vi "ActionVIOnCompile.vi"(8 "error in (no error)":errorcluster, 11 "Device Item Ref in":T1 format="%.0x") -> (0 "error out":errorcluster)   [LabVIEW 2021, in "FPGA Addon System Explorer.lvlib"]
uses:
  FPGA Addon System Explorer.lvlib
  <vilib>/NI VeriStand/Custom Device API/Custom Device Item Ref.ctl
  <vilib>/NI VeriStand/Custom Device API/Data Access Type.ctl
  Addon Shared/Types/FG Action.ctl
  Addon Shared/Types/Compiled.Settings.ctl
  Addon Shared/Types/Compiled.RegisterSettings.ctl
  Addon Shared/Types/Scalar Type.ctl
  Addon Shared/Types/Register Information.ctl
  Addon Shared/Types/FPGA Addon Data Type.ctl
  <vilib>/NI VeriStand/Custom Device API/Block Data Reference.ctl
  <vilib>/NI VeriStand/Custom Device API/Data Reference.ctl
  Addon Shared/Types/Compiled.DMASettings.ctl
  Addon Shared/Types/DMA Settings.ctl
  Addon Shared/Types/Delacing Scheme.ctl
  Addon Shared/Types/DMA Acquisition Mode.ctl
  <vilib>/NI VeriStand/Custom Device API/Waveform Data Reference.ctl
  Addon Shared/Types/FPGA Settings.ctl
  <vilib>/NI VeriStand/Custom Device API/Custom Device Target Type.ctl
  Addon Shared/SubVIs/Constants.vi
  <vilib>/NI VeriStand/Custom Device API/NI VeriStand - Get Item Property.vi
  <vilib>/NI VeriStand/Custom Device API/Get Item Property (Path).vi
  <vilib>/NI VeriStand/Custom Device API/Get Item Property (String).vi
  <vilib>/NI VeriStand/Custom Device API/Get Item Property (Boolean).vi
  <vilib>/NI VeriStand/Custom Device API/Set Item Property (Path).vi
  <vilib>/NI VeriStand/Custom Device API/Set Item Property (String).vi
  <vilib>/NI VeriStand/Custom Device API/Set Item Property (Boolean).vi
  <vilib>/NI VeriStand/Custom Device Tools/Custom Device Utility Library/NI VeriStand - Search for Item.vi
  <vilib>/NI VeriStand/Custom Device Tools/Custom Device Utility Library/NI VeriStand - Search for Item by GUID.vi
  SubVIs/Get Scalar Datatypes and Refs.vi
  <vilib>/NI VeriStand/Custom Device API/Set Item Property (Variant).vi
  <vilib>/NI VeriStand/Custom Device API/Custom Device API.lvlib
  Addon Shared/FPGA Addon Shared.lvlib
  <vilib>/NI/NIVS Inline Async API/_Data Access System Explorer/Data Access System Explorer.lvlib
  <vilib>/NI VeriStand/Custom Device Tools/Custom Device Utility Library/Custom Device Utility Library.lvlib
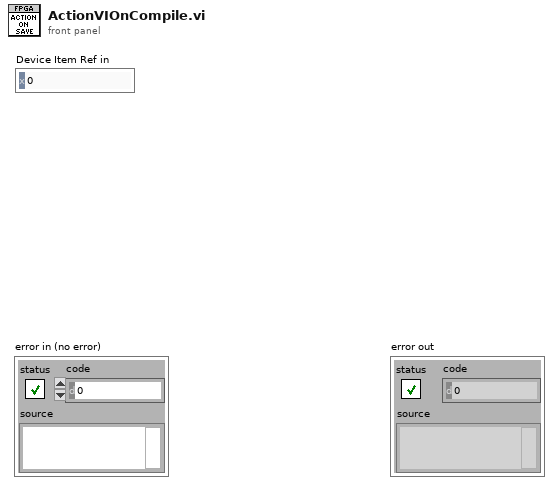
[diagram p1: front panel]
types:
  T1 = typedef "Custom Device API.lvlib/Custom Device Item Ref.ctl" = u64
  T2 = enum16{"Output/Write", "Input/Read", "Input/ReadWrite"}
  T3 = typedef "FPGA Addon Shared.lvlib/Compiled.Settings.ctl" = cluster{"Name":string, "IncomingRegisters.Settings":T4[], "IncomingRegisters.Refs":cluster{"Refs":T8[], "Values":dbl[]}, "OutgoingRegisters.Settings":T4[], "OutgoingRegisters.Refs":cluster{"Refs":T8[], "Values":dbl[]}, "Incoming.Size":i32, "Outgoing.Size":i32, "IncomingDMA.Settings":T10[], "OutgoingDMA.Settings":T10[], "FPGA.Settings":T15, "Target.Type":T16}
  T4 = typedef "FPGA Addon Shared.lvlib/Compiled.RegisterSettings.ctl" = cluster{"Scalar Type":T5, "Index":i32, "Length":i32, "Register":T6}
  T5 = typedef "FPGA Addon Shared.lvlib/Scalar Type.ctl" = enum16{"Standard", "Bitpacked"}
  T6 = typedef "FPGA Addon Shared.lvlib/Register Information.ctl" = cluster{"Name":string, "Data Type":T7, "Default Value":variant, "Attributes":variant}
  T7 = typedef "FPGA Addon Shared.lvlib/FPGA Addon Data Type.ctl" = enum8{"<Null>", "I8", "I16", "I32", "I64", "U8", "U16", "U32", "U64", "SGL", "Boolean", "Analog PWM In Settings", "Analog PWM In", "Digital PWM In Settings", "Digital PWM In", "Digital PWM Out", "Sine Out", "FXP", "FXP+/-24.5", "FXP+/-16.5", "FXP+/-32.8", "FXP+/-64.32", "FXP+/-16.7", "FXP+/-20.5", "FXP+/-27.5", "FXP+/-32.16", "FXP+16.3", "FXP+18.3", "Digital Static In", "Digital Static Out", "Digital Static In Settings", "Digital WSS Out", "Quad Encoder Settings", "Quad Encoder In", "Group"}
  T8 = typedef "Custom Device API.lvlib/Block Data Reference.ctl" = cluster{"Data Reference":T9, "Offset":u64, "Length":u64}
  T9 = typedef "Custom Device API.lvlib/Data Reference.ctl" = i32
  T10 = typedef "FPGA Addon Shared.lvlib/Compiled.DMASettings.ctl" = cluster{"Name":string, "Data Type":T7, "DMA.Settings":T11, "DMA.VSRefs":T14[]}
  T11 = typedef "FPGA Addon Shared.lvlib/DMA Settings.ctl" = cluster{"Number of Channels":u8, "Delacing Scheme":T12, "Update Rate":u32, "dt":dbl, "Mode":T13, "Number of Samples":u32, "DMA Host Buffer":u32}
  T12 = typedef "FPGA Addon Shared.lvlib/Delacing Scheme.ctl" = enum8{"Interleaved", "Bitpacked"}
  T13 = typedef "FPGA Addon Shared.lvlib/DMA Acquisition Mode.ctl" = enum8{"Continuous", "Triggered Finite"}
  T14 = typedef "Custom Device API.lvlib/Waveform Data Reference.ctl" = i32
  T15 = typedef "FPGA Addon Shared.lvlib/FPGA Settings.ctl" = cluster{"Bitfile path":path, "RIO Device Address":string, "Group":bool}
  T16 = typedef "Custom Device API.lvlib/Custom Device Target Type.ctl" = enum16{"PharLap", "VxWorks", "Windows", "Linux_32_ARM", "Linux_x64"}
  T17 = typedef "Custom Device API.lvlib/Data Access Type.ctl" = enum16{"Read", "Write"}
  T18 = typedef "FPGA Addon Shared.lvlib/FG Action.ctl" = enum8{"GET", "SET"}
  T19 = cluster{"Name":string, "Type":enum16{"Output/Write", "Input/Read", "Input/ReadWrite"}, "VS Refs":T1[]}
  T20 = typedef "Custom Device API.lvlib/Custom Device Item Info.ctl" = cluster{"Name":string, "Is Channel":bool, "GUID":string, "Is Waveform":bool}
  T21 = cluster{"Name":string, "Type":enum16{"Output/Write", "Input/Read", "Input/ReadWrite"}, "VS Refs":T1[]}[]
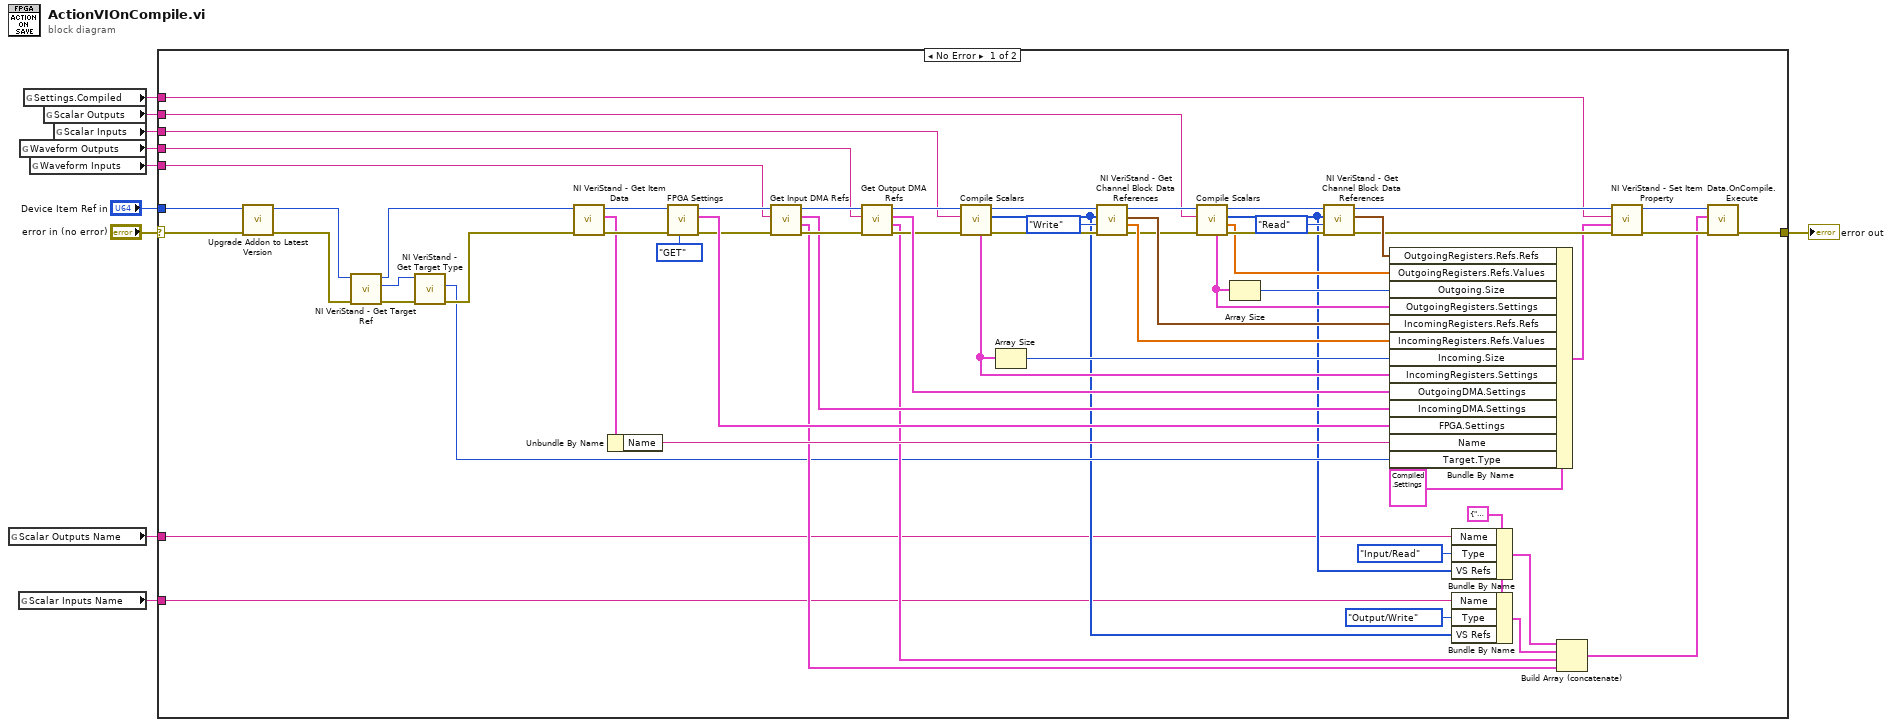
[diagram p0: block diagram]
diagram:
  n1 = global read "Constants.vi" "Scalar Outputs Name"() -> (w1:string)
  n2 = global read "Constants.vi" "Scalar Inputs Name"() -> (w2:string)
  n3 = global read "Constants.vi" "Waveform Outputs"() -> (w6:string)
  n4 = global read "Constants.vi" "Settings.Compiled"() -> (w3:string)
  n5 = global read "Constants.vi" "Waveform Inputs"() -> (w7:string)
  n6 = global read "Constants.vi" "Scalar Outputs"() -> (w4:string)
  n7 = global read "Constants.vi" "Scalar Inputs"() -> (w5:string)
  n8 = case shown="No Error" "error in (no error)" {
    selector: "error in (no error)" -> [w23 w74]
    tunnel: [w32 w74] -> w9
    tunnel: "Device Item Ref in" -> [w22 _]
    tunnel: w7 -> [w42 _]
    tunnel: w6 -> [w41 _]
    tunnel: w5 -> [w40 _]
    tunnel: w4 -> [w39 _]
    tunnel: w3 -> [w36 _]
    tunnel: w2 -> [w15 _]
    tunnel: w1 -> [w14 _]
    frame No Error {
      w11 = T19 {"Name"="", "Type"=enum."Output/Write", "VS Refs"=[]} ("Refs")
      n9 = call "Upgrade Addon to Latest Version.vi"("error in (no error)"=w23, "Device Item Ref in in"=w22) -> ("error out"=w21:errorcluster, "Device Item Ref out"=w20:T1)  [unwired: 8 in]
      n10 = call <vilib>:"NI VeriStand - Get Target Ref.vi"("error in"=w21, "Item Ref in"=w20) -> ("error out"=w29:errorcluster, "Target Ref"=w28:T1, "Item Ref out"=w26:T1)  [unwired: 6 in, 1 out]
      n11 = call <vilib>:"NI VeriStand - Get Target Type.vi"("error in (no error)"=w29, "Item Ref in"=w28) -> ("error out"=w27:errorcluster, "Target Type"=w25:T16)  [unwired: 7 in, 1 out]
      n12 = call <vilib>:"NI VeriStand - Get Item Data.vi"("error in (no error)"=w27, "Item Ref in"=w26) -> ("error out"=w71:errorcluster, "Item Info"=w59:T20, "Item Ref out"=w70:T1)  [unwired: 6 in, 1 out]
      n13 = Unbundle By Name(w59) -> ("Name"=w60:string)
      n14 = call "FPGA Settings.vi"("Action"=FG_Action."GET", "error in (no error)"=w71, "Item Ref"=w70) -> ("error out"=w72:errorcluster, "FPGA Settings"=w73:T15, "Item Ref out"=w61:T1)  [unwired: 6 in]
      n15 = call "Get Input DMA Refs.vi"("error in (no error)"=w72, "Item GUID"=w42, "Section Ref in"=w61) -> ("error out"=w63:errorcluster, "Refs"=w35:T21, "DMA Settings"=w62:T10[], "Section Ref out"=w65:T1)  [unwired: 5 in]
      n16 = call "Get Output DMA Refs.vi"("error in (no error)"=w63, "Item GUID"=w41, "Section Ref in"=w65) -> ("error out"=w64:errorcluster, "Refs"=w34:T21, "DMA"=w67:T10[], "Section Ref out"=w66:T1)  [unwired: 5 in]
      n17 = call "Compile Scalars.vi"("error in (no error)"=w64, "Item GUID"=w40, "Section Ref in"=w66) -> ("error out"=w46:errorcluster, "VS Ref"=w16:T1[], "Section Ref out"=w45:T1, "Registers Ref"=w68:T4[])  [unwired: 4 in, 1 out]
      n18 = Array Size(array=w68) -> (size(s)=w57:i32)
      n19 = call <vilib>:"NI VeriStand - Get Channel Block Data References.vi"("error in (no error)"=w46, "Access"=Data_Access_Type."Write", "Channel Refs"=w16, "Device Ref in"=w45) -> ("error out"=w47:errorcluster, "Values Array"=w58:dbl[], "Block Data Refs"=w54:T8[], "Device Ref out"=w48:T1)  [unwired: 4 in]
      n20 = call "Compile Scalars.vi"("error in (no error)"=w47, "Item GUID"=w39, "Section Ref in"=w48) -> ("error out"=w50:errorcluster, "Default Values"=w24:dbl[], "VS Ref"=w17:T1[], "Section Ref out"=w51:T1, "Registers Ref"=w69:T4[])  [unwired: 4 in]
      n21 = Array Size(array=w69) -> (size(s)=w56:i32)
      n22 = call <vilib>:"NI VeriStand - Get Channel Block Data References.vi"("error in (no error)"=w50, "Access"=Data_Access_Type."Read", "Channel Refs"=w17, "Device Ref in"=w51) -> ("error out"=w43:errorcluster, "Block Data Refs"=w55:T8[], "Device Ref out"=w37:T1)  [unwired: 4 in, 1 out]
      n23 = Bundle By Name(cluster=T3 {"Name"="", "IncomingRegisters.Settings"=[], "IncomingRegisters.Refs"={"Refs"=[], "Values"=[]}, "OutgoingRegisters.Settings"=[], "OutgoingRegisters.Refs"={"Refs"=[], "Values"=[]}, "Incoming.Size"=0, "Outgoing.Size"=0, "IncomingDMA.Settings"=[], "OutgoingDMA.Settings"=[], "FPGA.Settings"={"Bitfile path"=path "", "RIO Device Address"="", "Group"=FALSE}, "Target.Type"=enum."PharLap"}, "OutgoingRegisters.Refs.Refs"=w55, "OutgoingRegisters.Refs.Values"=w24, "Outgoing.Size"=w56, "OutgoingRegisters.Settings"=w69, "IncomingRegisters.Refs.Refs"=w54, "IncomingRegisters.Refs.Values"=w58, "Incoming.Size"=w57, "IncomingRegisters.Settings"=w68, "OutgoingDMA.Settings"=w67, "IncomingDMA.Settings"=w62, "FPGA.Settings"=w73, "Name"=w60, "Target.Type"=w25) -> (w38:T3)
      n24 = Bundle By Name(cluster=w11, "Name"=w14, "Type"=T2."Input/Read", "VS Refs"=w17) -> (w18:T19)
      n25 = Bundle By Name(cluster=w11, "Name"=w15, "Type"=T2."Output/Write", "VS Refs"=w16) -> (w19:T19)
      n26 = Build Array (concatenate)(w18, w19, w34, w35) -> (w30:T21)
      n27 = call-poly <vilib>:"NI VeriStand - Set Item Property.vi"("error in (no error)"=w43, "Value"=w38, "Property Name"=w36, "Item Ref in"=w37) -> ("error out"=w33:errorcluster, "Item Ref out"=w31:T1)  [unwired: 5 in, 1 out]
      n28 = call <vilib>:"Data.OnCompile.Execute.vi"("error in"=w33, "VS Ref Groups"=w30, "Custom Device Ref"=w31) -> ("error out"=w32:errorcluster)  [unwired: 7 in, 1 out]
    }
    frame Error {
    }
  }
  "error out" <- w9
